vi "adjust.vi"(8 "error in (no error)":errorcluster, 11 "GenericEmissionSensor in":refnum<class "DetectorDL090603DAQmxOnOff.lvclass">) -> (0 "error out":errorcluster, 3 "GenericEmissionSensor out":refnum<class "DetectorDL090603DAQmxOnOff.lvclass">)   [LabVIEW 2010, in "DetectorDL090603DAQmxOnOff.lvclass"]
uses:
  DetectorDL090603DAQmxOnOff.lvclass
  DetectorDL090603DAQmxOnOff.lvclass/DetectorDL090603DAQmxOnOff.ctl
panel:
  in  "done":bool
  in  "Voltage":dbl[unit](slide) scale=0.0..10.0
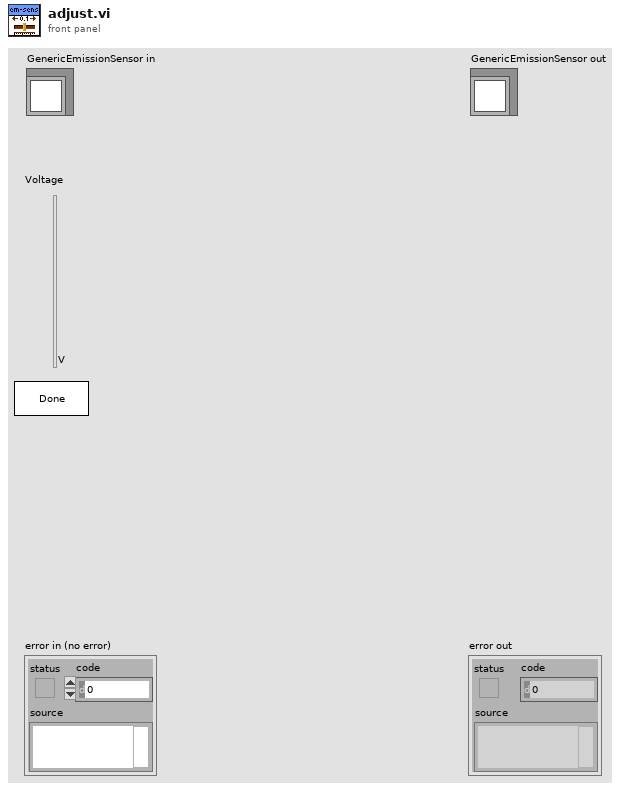
[diagram p1: front panel]
types:
  T1 = typedef "GenericDetector.lvclass/status_enum.ctl" = enum16{"disabled", "enabled"}
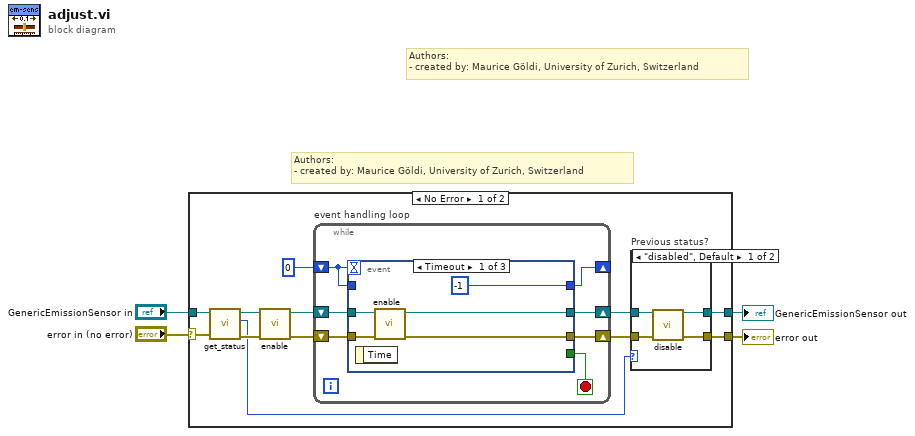
[diagram p0: block diagram]
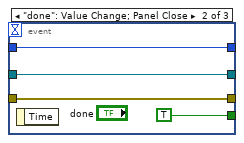
[diagram p3: hidden frame]
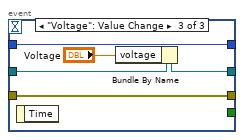
[diagram p4: hidden frame]
diagram:
  # "Authors: \n- created by: Maurice Göldi, University of Zurich, Switzerland"
  # "Authors: \n- created by: Maurice Göldi, University of Zurich, Switzerland"
  n1 = case shown="No Error" "error in (no error)" {
    selector: "error in (no error)" -> [w15 w45]
    tunnel: [w7 w45] -> w3
    tunnel: "GenericEmissionSensor in" -> [w13 w44]
    tunnel: [w5 w44] -> w1
    frame No Error {
      n2 = call-dynamic "get_status.vi"("error in (no error)"=w15, "GenericEmissionSensor.lvclass in"=w13) -> ("error out"=w14:errorcluster, "status"=w9:T1, "GenericEmissionSensor.lvclass out"=w12:refnum<class "DetectorDL090603DAQmxOnOff.lvclass">)  [unwired: 7 in]
      n3 = call-dynamic "enable.vi"("error in (no error)"=w14, "DL090603DAQmxOnOffEmissionSensor in"=w12) -> ("error out"=w11:errorcluster, "DL090603DAQmxOnOffEmissionSensor out"=w10:refnum<class "DetectorDL090603DAQmxOnOff.lvclass">)  [unwired: 8 in]
      n4 = while "event handling loop" {
        shift-right: [w29] -> _
        shift-left: 0 -> [w23]
        shift-right: [w26] -> w8
        shift-left: w11 -> [w28]
        shift-right: [w25] -> w6
        shift-left: w10 -> [w27]
        stop <- w24 stop-if-true
        n5 = event shown="[0] Timeout" {
          selector: _ -> [_ _ _]
          dyn-events: _ -> [_ _ _]
          timeout: w23 -> [_ _ _]
          tunnel: w23 -> [_ w35 w39]
          tunnel: [-1 w35 w39] -> w29
          tunnel: w28 -> [w33 w38 w43]
          tunnel: w27 -> [w32 w37 w42]
          tunnel: [w31 w38 w43] -> w26
          tunnel: [w30 w37 w41] -> w25
          tunnel: [_ TRUE _] -> w24
          event Timeout {
            n6 = event-data() -> ()  [unwired: 1 in, 1 out]
            n7 = call-dynamic "enable.vi"("error in (no error)"=w33, "DL090603DAQmxOnOffEmissionSensor in"=w32) -> ("error out"=w31:errorcluster, "DL090603DAQmxOnOffEmissionSensor out"=w30:refnum<class "DetectorDL090603DAQmxOnOff.lvclass">)  [unwired: 8 in]
          }
          event "done": Value Change; Panel Close {
            n8 = event-data() -> ()  [unwired: 1 in, 1 out]
          }
          event "Voltage": Value Change {
            n9 = event-data() -> ()  [unwired: 1 in, 1 out]
            n10 = Bundle By Name(cluster=w42, "voltage"="Voltage") -> (w41:refnum<class "DetectorDL090603DAQmxOnOff.lvclass">)
          }
        }
      }
      n11 = case "Previous status?" shown="\"disabled\", Default" w9 {
        tunnel: w8 -> [w20 w21]
        tunnel: [w19 w21] -> w7
        tunnel: w6 -> [w18 w22]
        tunnel: [w17 w22] -> w5
        frame "disabled", Default {
          n12 = call-dynamic "disable.vi"("error in (no error)"=w20, "DL090603DAQmxOnOffEmissionSensor in"=w18) -> ("error out"=w19:errorcluster, "DL090603DAQmxOnOffEmissionSensor out"=w17:refnum<class "DetectorDL090603DAQmxOnOff.lvclass">)  [unwired: 8 in]
        }
        frame "enabled" {
        }
      }
    }
    frame Error {
    }
  }
  "error out" <- w3
  "GenericEmissionSensor out" <- w1
